vi "My Current source Initialization (SubVI).vi"(6 "Output Low Connection":T1, 7 "Current level":dbl format="%#_13g", 8 "error in (no error)":errorcluster, 9 "Current Range In":T2={"Auto Range?"=TRUE, "Man / Selected\nRange"=enum."2nA"}, 10 "Voltage limit (V)":dbl format="%#_13g", 11 "VISA Refnum in":refnum<visa-resource-name>) -> (0 "error out":errorcluster, 3 "VISA Refnum out":refnum<visa-resource-name>)   [LabVIEW 2025, in "My Current Source.lvlib"]
uses:
  My Current Source.lvlib
  KE622x -- Current Range.ctl
  KE622x -- Current Ranges.ctl
  KE622x -- Output Low Connection.ctl
  KE622x -- Instrument Type.ctl
  KE622x -- On Off Control.ctl
  KE6221 -- Output Response.ctl
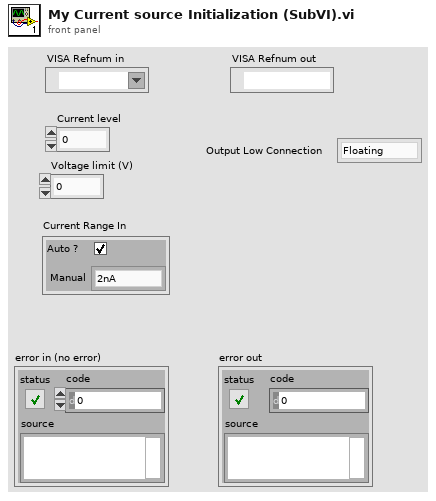
[diagram p1: front panel]
types:
  T1 = typedef "My Current Source.lvlib/KE622x -- Output Low Connection.ctl" = enum16{"Floating", "Earth Ground"}
  T2 = typedef "My Current Source.lvlib/KE622x -- Current Range.ctl" = cluster{"Auto Range?":bool, "Man / Selected\nRange":T3}
  T3 = typedef "My Current Source.lvlib/KE622x -- Current Ranges.ctl" = enum16{"2nA", "20nA", "200nA", "2uA", "20uA", "200uA", "2mA", "20mA", "100mA"}
  T4 = typedef "My Current Source.lvlib/KE6221 -- Output Response.ctl" = enum16{"Fast", "Slow"}
  T5 = typedef "My Current Source.lvlib/KE622x -- On Off Control.ctl" = enum16{"Off", "On"}
  T6 = typedef "My Current Source.lvlib/KE622x -- Instrument Type.ctl" = enum16{"KE6220", "KE6221"}
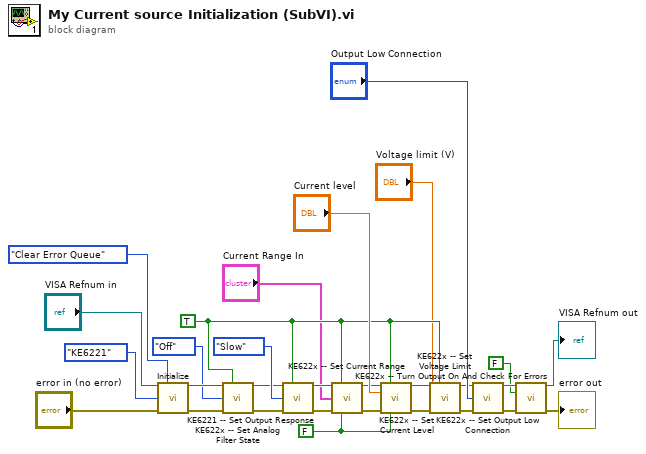
[diagram p0: block diagram]
diagram:
  w18 = TRUE ("Check For SCPI Errors? (T)")
  w15 = FALSE ("Read Back Set Values? (T)")
  n1 = call "Initialize.vi"("VISA resource name"="VISA Refnum in", "Error Queue Option"=enum16{"Clear Error Queue", "Error Query"}."Clear Error Queue", "Instrument Type"=KE622x_--_Instrument_Type."KE6221", "error in (no error)"="error in (no error)") -> ("VISA resource name out"=w6:refnum<visa-resource-name>, "error out"=w7:errorcluster)  [unwired: 10 in]
  n2 = call "KE622x -- Set Analog Filter State.vi"("Resource In"=w6, "Check For SCPI Errors? (T)"=w18, "Analog Filter State"=KE622x_--_On_Off_Control."Off", "error in (no error)"=w7) -> ("Resource Out (dupl)"=w8:refnum<visa-resource-name>, "error out"=w10:errorcluster)  [unwired: 10 in]
  n3 = call "KE6221 -- Set Output Response.vi"("Resource In"=w8, "Check For SCPI Errors? (T)"=w18, "KE6221 Output Response"=KE6221_--_Output_Response."Slow" ("Output Response"), "error in (no error)"=w10) -> ("Resource Out (dupl)"=w12:refnum<visa-resource-name>, "error out"=w11:errorcluster)  [unwired: 10 in]
  n4 = call "KE622x -- Set Current Range.vi"("Resource In"=w12, "Check For SCPI Errors? (T)"=w18, "Current Range In"="Current Range In", "error in (no error)"=w11, "Read Back Set Values? (T)"=w15) -> ("Resource Out (dupl)"=w13:refnum<visa-resource-name>, "error out"=w14:errorcluster)  [unwired: 8 in, 1 out]
  n5 = call "KE622x -- Set Current Level.vi"("Resource In"=w13, "Check For SCPI Errors? (T)"=w18, "Current value"="Current level", "error in (no error)"=w14, "Read Back Set Value? (T)"=w15) -> ("Resource Out (dupl)"=w16:refnum<visa-resource-name>, "error out"=w17:errorcluster)  [unwired: 8 in, 1 out]
  n6 = call "KE622x -- Set Voltage Limit.vi"("Resource In"=w16, "Check For SCPI Errors? (T)"=w18, "Voltage limit (V)"="Voltage limit (V)", "error in (no error)"=w17) -> ("Resource Out (dupl)"=w21:refnum<visa-resource-name>, "error out"=w22:errorcluster)  [unwired: 10 in]
  n7 = call "KE622x -- Set Output Low Connection.vi"("Resource In"=w21, "Output Low Connection"="Output Low Connection", "error in (no error)"=w22) -> ("Resource Out (dupl)"=w24:refnum<visa-resource-name>, "error out"=w23:errorcluster)  [unwired: 11 in]
  n8 = call "KE622x -- Turn Output On And Check For Errors.vi"("Resource In"=w24, "Turn Off Output If Compliance?"=FALSE ("Turn Off Output If Voltage Limit?"), "error in (no error)"=w23) -> ("Resource Out (dupl)"=→"VISA Refnum out":refnum<visa-resource-name>, "error out"=→"error out":errorcluster)  [unwired: 9 in, 2 out]
